vi "get tag names for lines.vi"(8 "error in (no error)":errorcluster, 9 "Lines in":T1[](array[typedef]), 10 "engine in":refnum<class "Engine Parent Editor Node.lvclass">, 11 "editor node in":refnum<class "module editor node.lvclass">) -> (0 "error out":errorcluster, 1 "Lines out":T1[](array[typedef]), 2 "engine out":refnum<class "Engine Parent Editor Node.lvclass">, 3 "editor node out":refnum<class "module editor node.lvclass">, 5 "tag names":string[](array[string]))   [LabVIEW 2014, in "Shared Memory editor node.lvclass"]
uses:
  Shared Memory editor node.lvclass
  module/configuration/Line.ctl
  <vilib>/NI/Tag Bus Module Framework/channel/TBM channel.lvclass
  <vilib>/NI/DCAF/Tag Editor Core/Configuration Editor/Classes/Module editor node/module editor node.lvclass
  <vilib>/NI/DCAF/Tag Editor Core/Configuration Editor/Classes/Engine Parent/Engine Parent Editor Node.lvclass
  module/configuration/Shared Memory configuration.lvclass
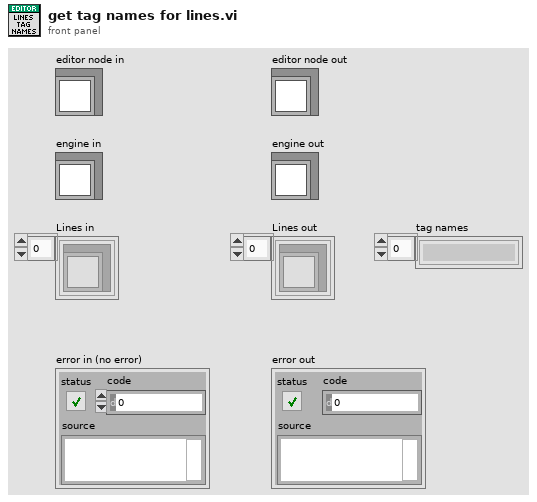
[diagram p1: front panel]
types:
  T1 = typedef "Shared Memory configuration.lvclass/Line.ctl" = cluster{"channel":refnum<class "TBM channel.lvclass">}
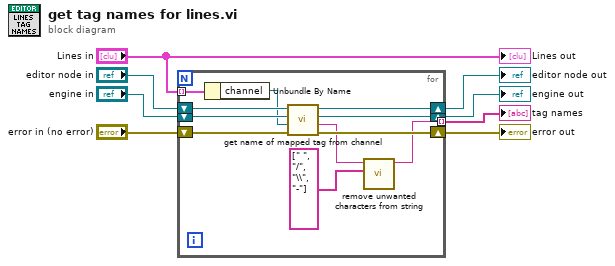
[diagram p0: block diagram]
diagram:
  n1 = for {
    tunnel: "Lines in" -> [w19] mode=indexing
    tunnel: [w9] -> w7 mode=indexing
    shift-right: [w17] -> w3
    shift-left: "engine in" -> [w18]
    shift-right: [w16] -> w4
    shift-left: "editor node in" -> [w15]
    shift-right: [w13] -> w1
    shift-left: "error in (no error)" -> [w12]
    n2 = Unbundle By Name(w19) -> ("channel"=w14:refnum<class "TBM channel.lvclass">)
    n3 = call "get name of mapped tag from channel.vi"("error in (no error)"=w12, "channel"=w14, "engine in"=w18, "editor node in"=w15) -> ("error out"=w13:errorcluster, "tag name"=w10:string, "engine out"=w17:refnum<class "Engine Parent Editor Node.lvclass">, "editor node out"=w16:refnum<class "module editor node.lvclass">)  [unwired: 4 in]
    n4 = call "remove unwanted characters from string.vi"("unwanted patterns/characters"=string[] [" ", "/", "\\", "-"], "string in"=w10) -> ("string out"=w9:string)  [unwired: 9 in]
  }
  "tag names" <- w7
  "editor node out" <- w4
  "engine out" <- w3
  "error out" <- w1
  "Lines out" <- "Lines in"
